vi "Sprinkler.vi"() -> ()   [LabVIEW 2013]
uses:
  Controls/Sprinkler State.ctl
  Controls/Read Write States.ctl
panel:
  in  "Zone Setup Array":cluster{"Zone Selector":string, "Timing":dbl}[](array[cluster])
  out "Controller Status":string
  out "Zone Indicators":T1
  in  "Water Pressure Sensor (%)":u32(slide) scale=0.0..100.0
  in  "Rain Sensor":bool
  in  "Run Selector":bool
  in  "Setup":bool
  in  "Start":bool
  in  "stop":bool
  # "Controls"
  # "Simulation Controls"
  # "Rain"
  # "No Rain"
  # "Continuous"
  # "Single"
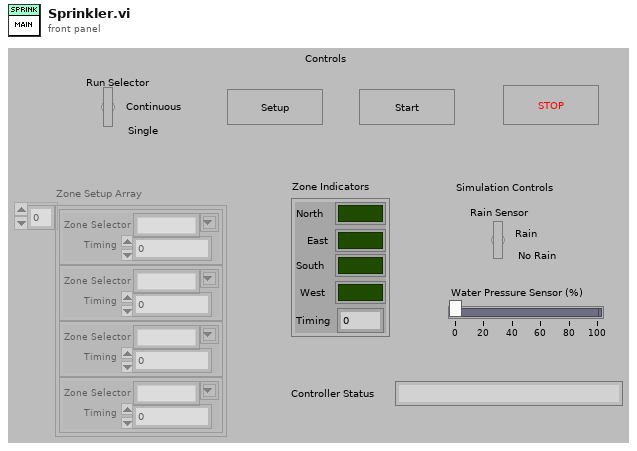
[diagram p1: front panel]
types:
  T1 = cluster{"North":bool, "East":bool, "South":bool, "West":bool, "Timing":u32}
  T2 = typedef "Sprinkler State.ctl" = enum16{"Initialize", "Main", "Stop"}
  T3 = enum8{"Enabled", "Disabled", "Disabled and Grayed Out"}
  T4 = typedef "Read Write States.ctl" = enum16{"Initialize", "Read", "Write", "Stop"}
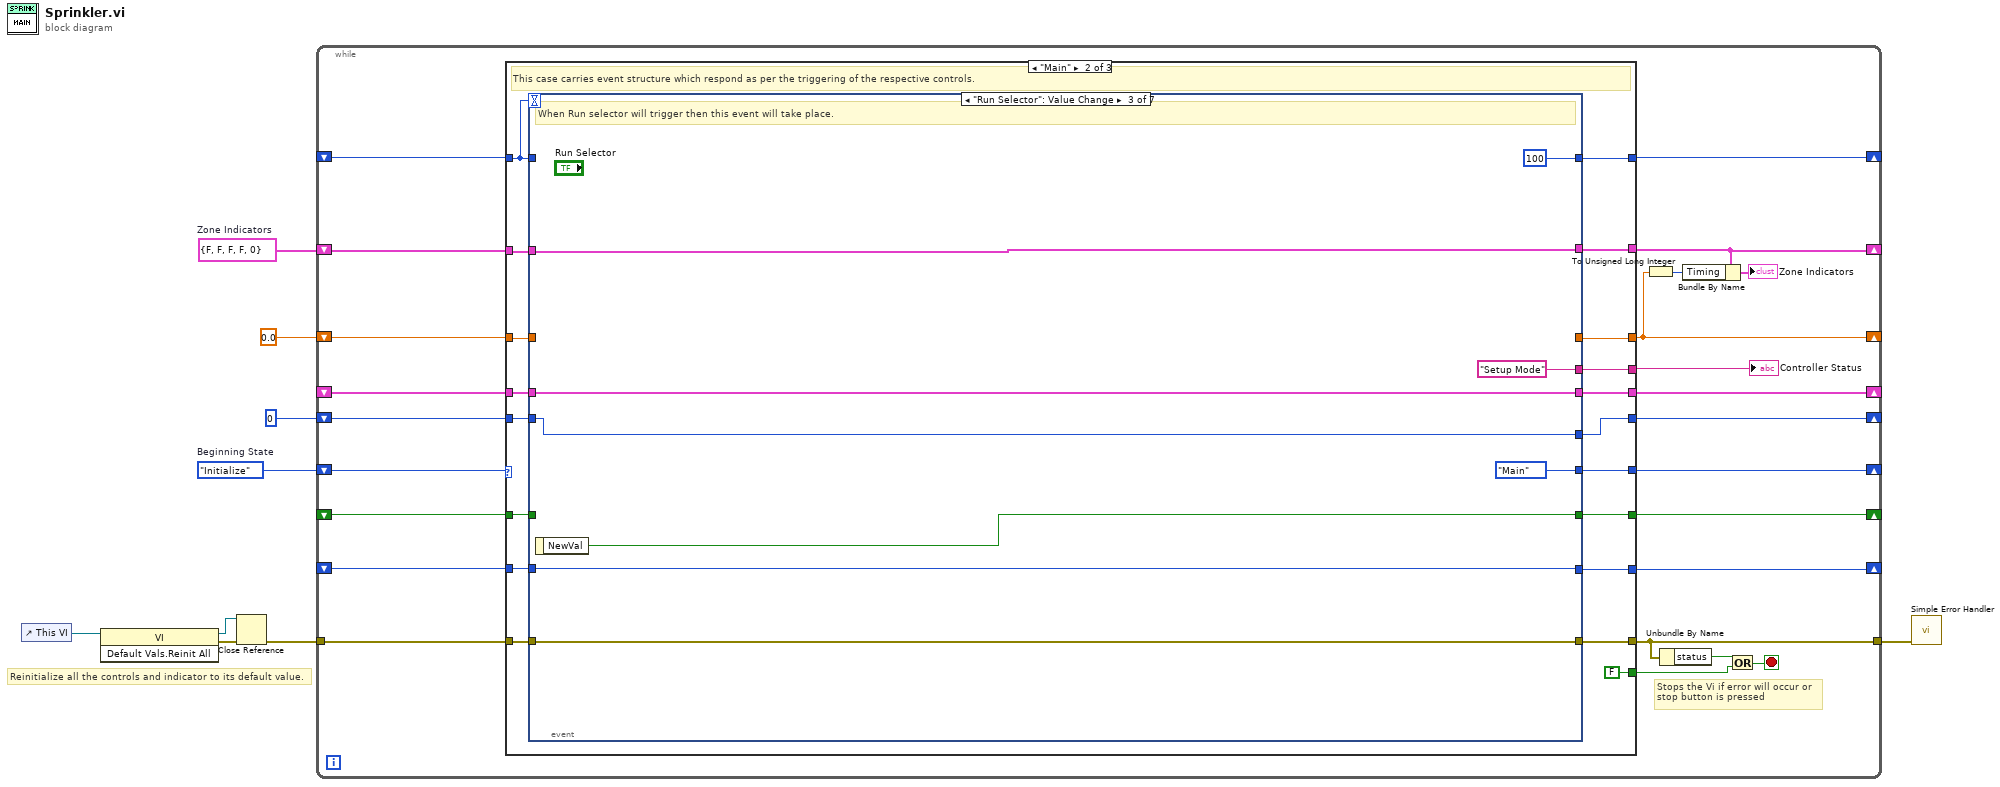
[diagram p0: block diagram]
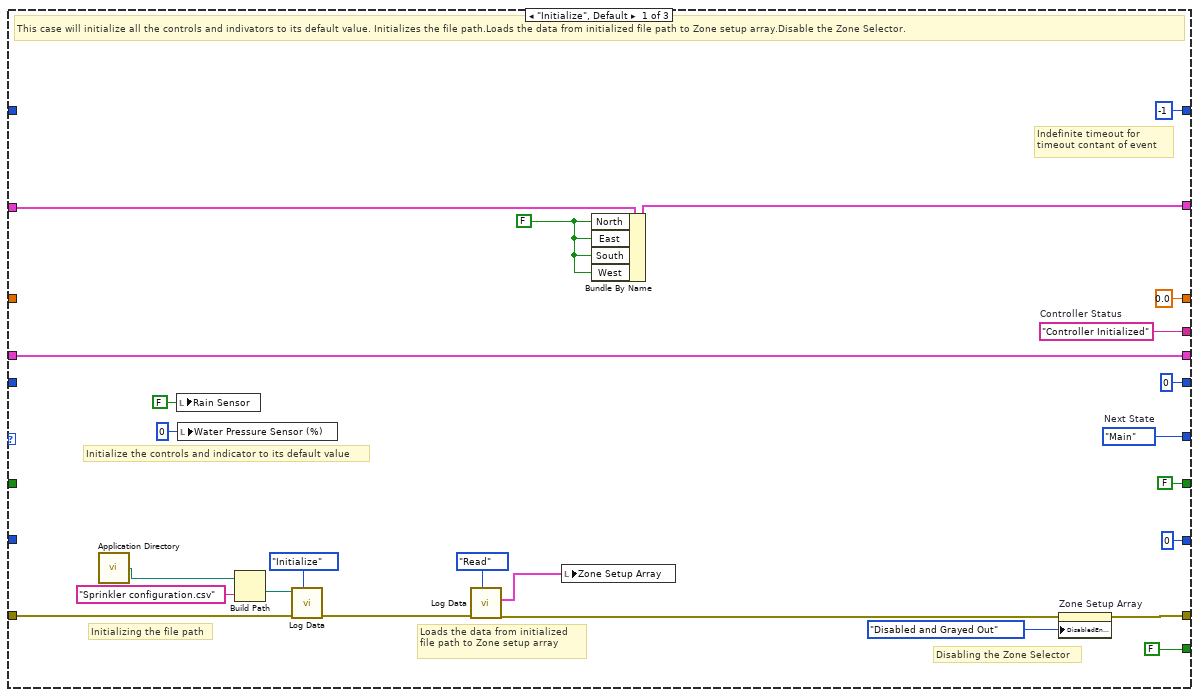
[diagram p2: hidden frame]
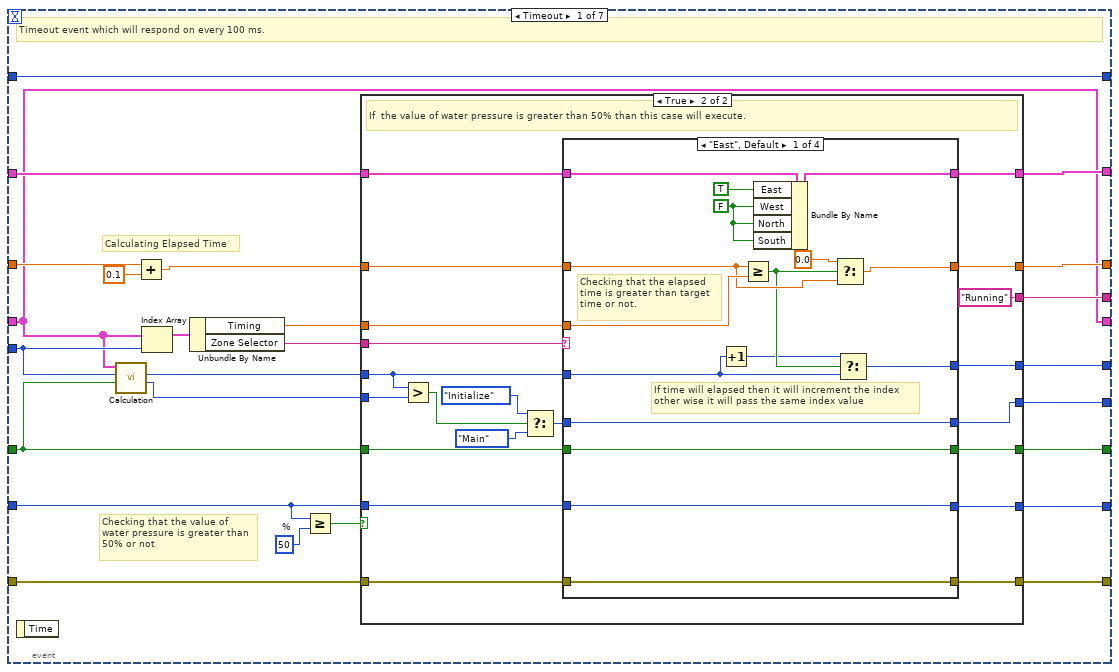
[diagram p3: hidden frame]
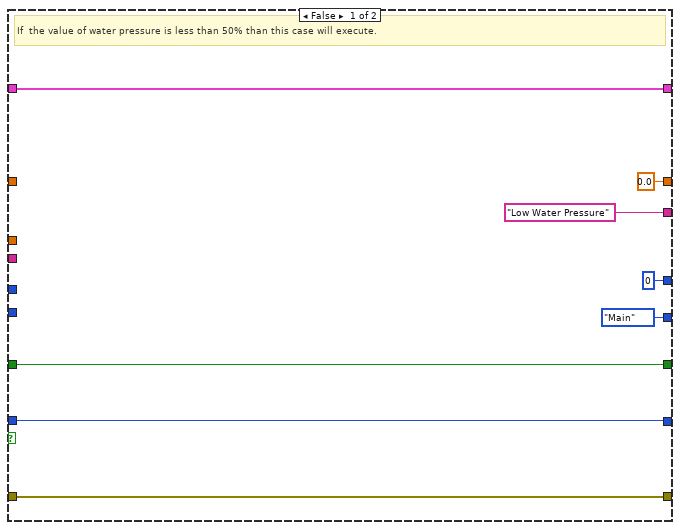
[diagram p4: hidden frame]
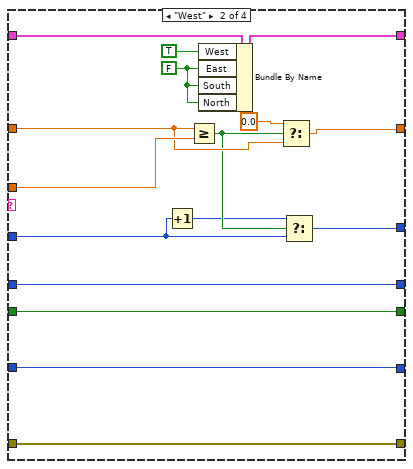
[diagram p5: hidden frame]
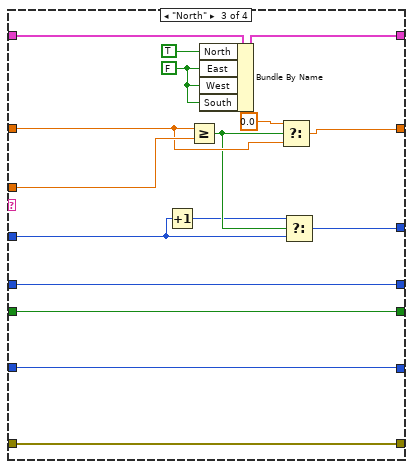
[diagram p6: hidden frame]
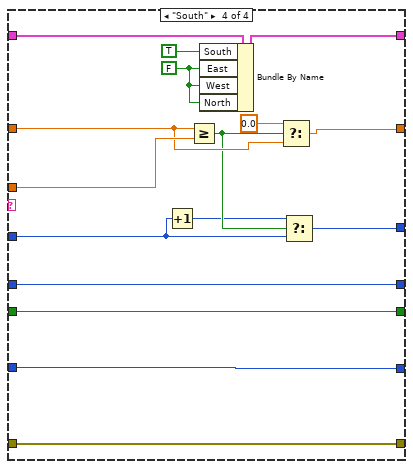
[diagram p7: hidden frame]
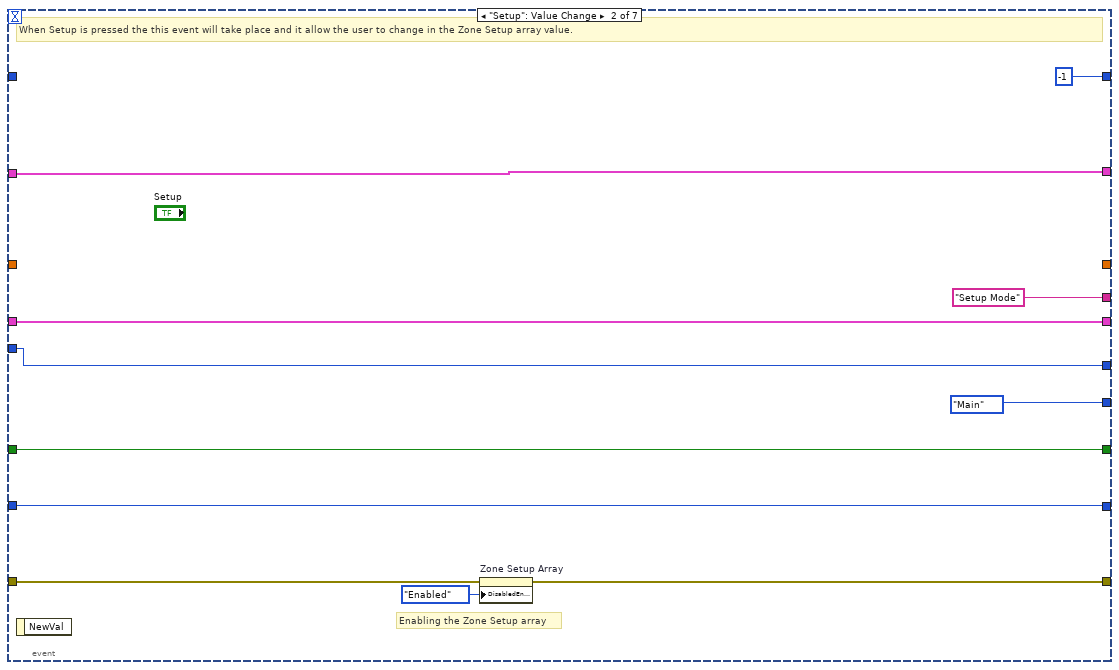
[diagram p8: hidden frame]
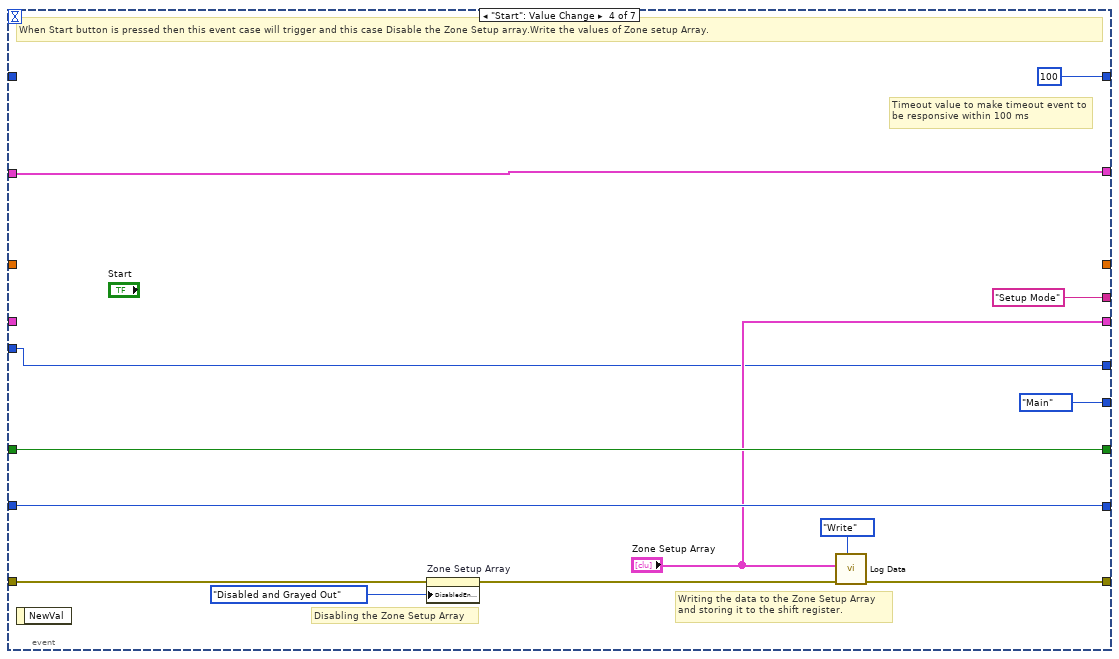
[diagram p9: hidden frame]
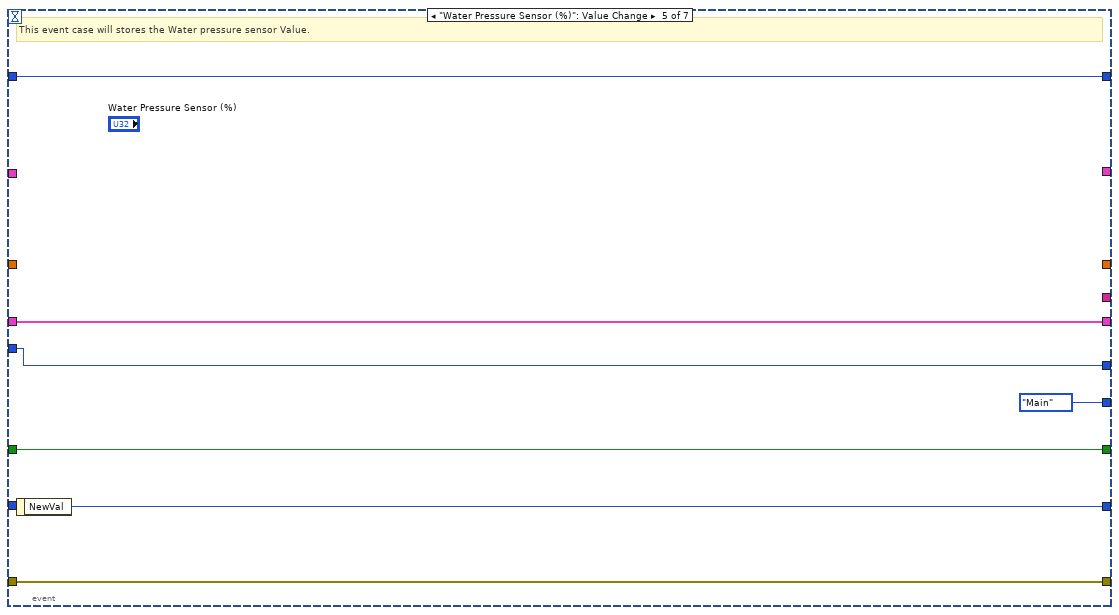
[diagram p10: hidden frame]
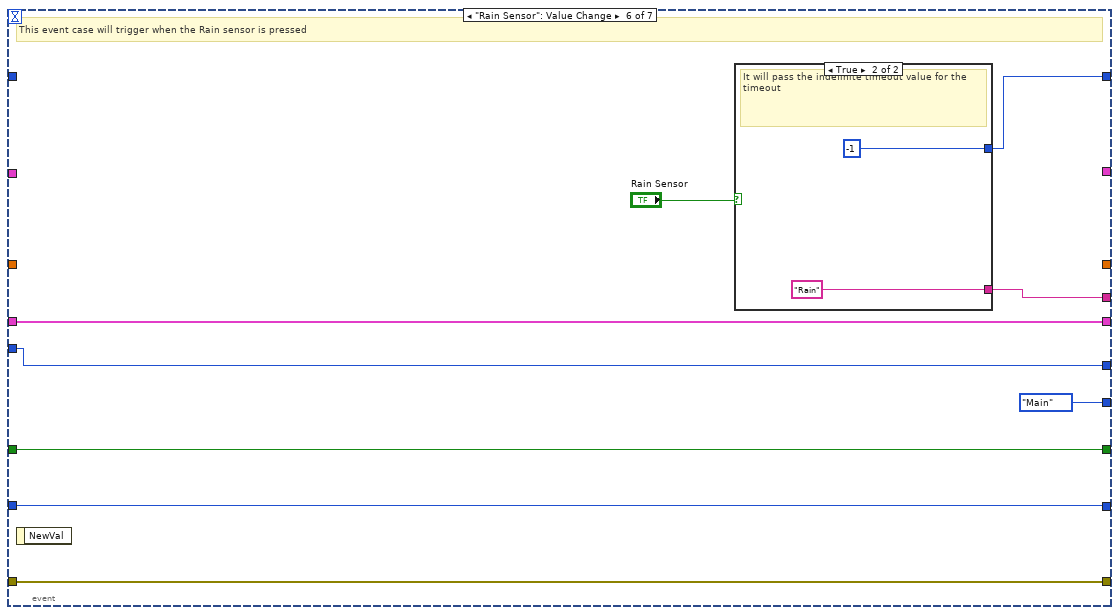
[diagram p11: hidden frame]
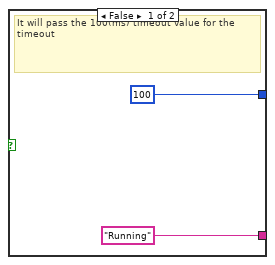
[diagram p12: hidden frame]
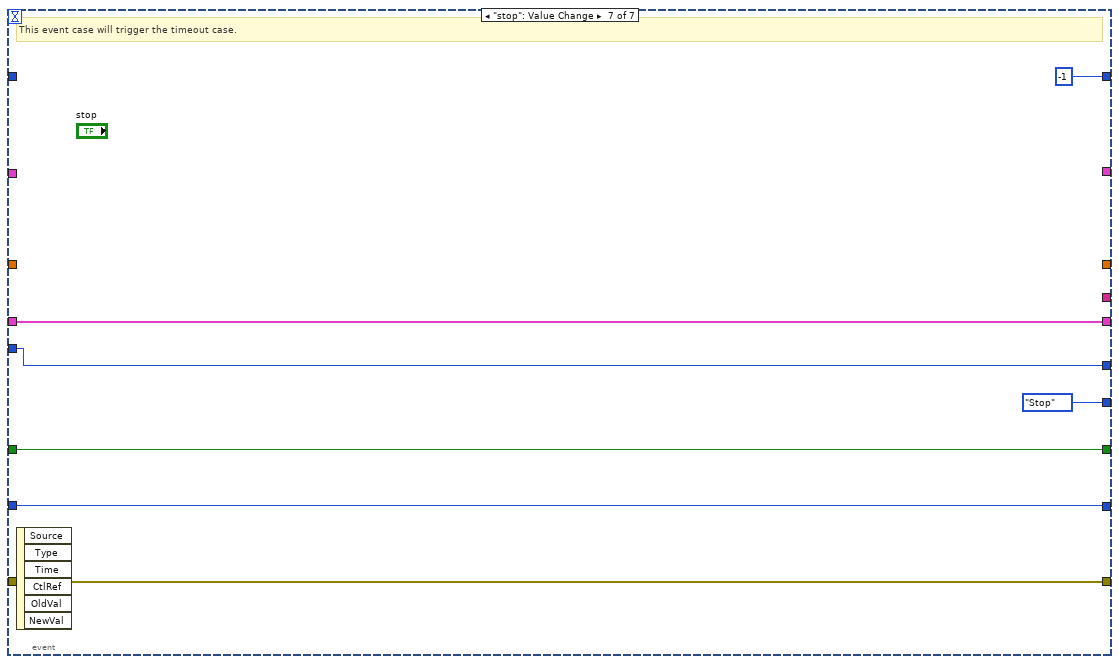
[diagram p13: hidden frame]
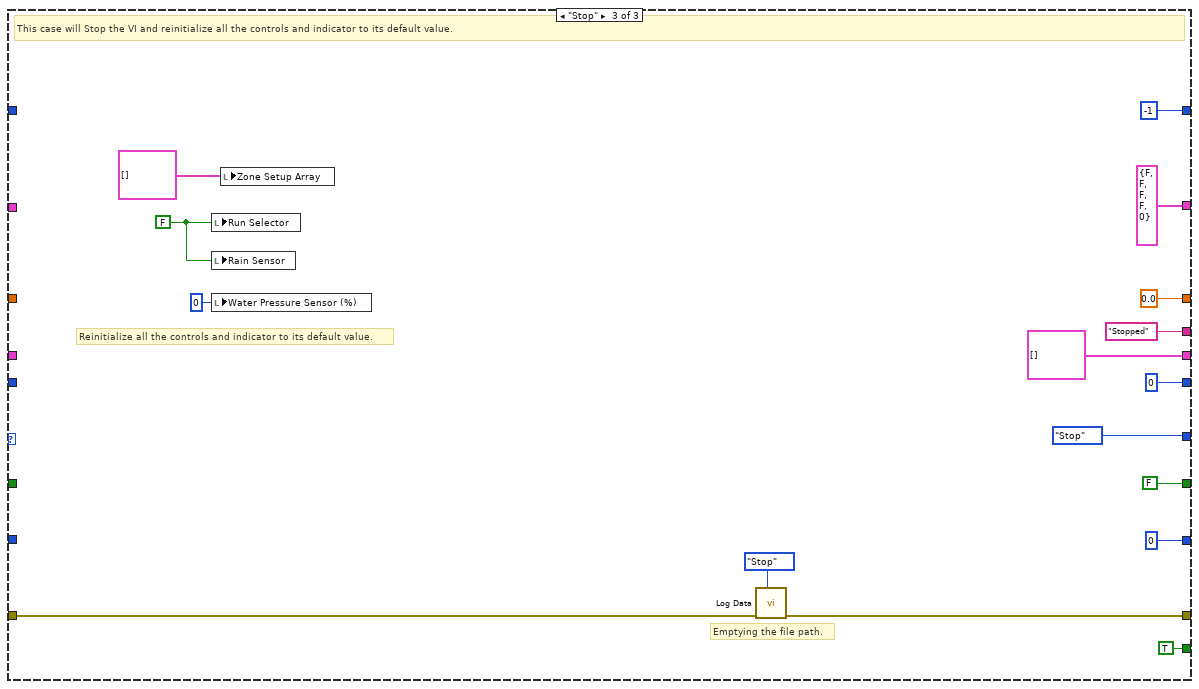
[diagram p14: hidden frame]
diagram:
  w4 = T1 {"North"=FALSE, "East"=FALSE, "South"=FALSE, "West"=FALSE, "Timing"=0}  # Zone Indicators
  w9 = Sprinkler_State."Initialize"  # Beginning State
  # "Reinitialize all the controls and indicator to its default value."
  n1 = control-ref of="This VI"() -> (w6:refnum<vi>)
  n2 = invoke class="VI" method="Default Vals.Reinit All"(reference=w6) -> (reference out=w7:refnum<vi>, error out=w8:errorcluster)  [unwired: 2 in, 1 out]
  n3 = Close Reference(reference=w7, error in (no error)=w8) -> (error out=w5:errorcluster)
  n4 = while {
    shift-right: [w32] -> _
    shift-left: w9 -> [w33]
    tunnel: w5 -> [w31]
    tunnel: [w27] -> w1
    shift-right: [w28] -> _
    shift-left: w4 -> [w29]
    shift-right: [w23] -> _
    shift-left: _ -> [w13]
    shift-right: [w22] -> _
    shift-left: _ -> [w21]
    shift-right: [w18] -> _
    shift-left: 0.0 -> [w20]
    shift-right: [w16] -> _
    shift-left: _ -> [w10]
    shift-right: [w14] -> _
    shift-left: 0 -> [w15]
    shift-right: [w12] -> _
    shift-left: _ -> [w11]
    stop <- w24 stop-if-true
    # "Stops the Vi if error will occur or stop button is pressed"
    n5 = case shown="\"Main\"" w33 {
      tunnel: [w58 w62 Sprinkler_State."Stop" ("Next State")] -> w32
      tunnel: w31 -> [w57 w76 w258]
      tunnel: [w39 w75 w257] -> w27
      tunnel: [w50 w74 "Stopped" ("Controller Status")] -> w30
      tunnel: [w36 w72 T1 {"North"=FALSE, "East"=FALSE, "South"=FALSE, "West"=FALSE, "Timing"=0} ("Zone Indicators")] -> w28
      tunnel: w29 -> [w49 w73 _]
      tunnel: [FALSE FALSE TRUE] -> w25
      tunnel: [FALSE ("NewVal") w71 FALSE ("NewVal")] -> w23
      tunnel: [-1 w70 -1] -> w22
      tunnel: w21 -> [_ w63 _]
      tunnel: w20 -> [_ w69 _]
      tunnel: [0.0 ("t") w68 0.0 ("t")] -> w18
      tunnel: [u32 0 ("NewVal") w67 u32 0 ("NewVal")] -> w16
      tunnel: w15 -> [_ w66 _]
      tunnel: [0 ("t") w65 0 ("t")] -> w14
      tunnel: w13 -> [_ w64 _]
      tunnel: [w37 w61 cluster{"Zone Selector":string, "Timing":dbl}[] [] ("Zone Setup Array")] -> w12
      tunnel: w11 -> [w37 w60 _]
      tunnel: w10 -> [_ w59 _]
      frame "Initialize", Default {
        w35 = FALSE ("North")
        w50 = "Controller Initialized"  # Controller Status
        w58 = Sprinkler_State."Main"  # Next State
        # "Indefinite timeout for \ntimeout contant of event"
        # "Disabling the Zone Selector"
        # "Loads the data from initialized file path to Zone setup array"
        # "Initializing the file path"
        # "Initialize the controls and indicator to its default value"
        # "This case will initialize all the controls and indivators to its default value. Initializes the file path.Loads the data from initialized file path to Zone setup array.Disable the Zone Selector."
        n6 = call <vilib>:"Application Directory.vi"() -> ("Application Directory"=w55:path)
        n7 = local write "Rain Sensor"(FALSE ("Rain Sensor")) -> ()
        n8 = local write "Water Pressure Sensor (%)"(u32 0 ("Water Pressure Sensor (%)")) -> ()
        n9 = Build Path(base path=w55, name or relative path="Sprinkler configuration.csv") -> (appended path=w53:path)
        n10 = call "Log Data.vi"("Command"=Read_Write_States."Initialize", "error in (no error)"=w57, "file path"=w53) -> ("error out"=w52:errorcluster)  [unwired: 7 in, 1 out]
        n11 = call "Log Data.vi"("Command"=Read_Write_States."Read", "error in (no error)"=w52) -> ("error out"=w40:errorcluster, "Array"=w38:cluster{"Zone Selector":string, "Timing":dbl}[])  [unwired: 8 in]
        n12 = local write "Zone Setup Array"(w38) -> ()
        n13 = Bundle By Name(cluster=w49, "North"=w35, "East"=w35, "South"=w35, "West"=w35) -> (w36:T1)
        n14 = property on="Zone Setup Array" class="Arr (strict)"(error in=w40, "DisabledEnum"=T3."Disabled and Grayed Out" ("Disabled")) -> (error out=w39:errorcluster)  [unwired: 1 in, 1 out]
      }
      frame "Main" {
        # "This case carries event structure which respond as per the triggering of the respective controls."
        n15 = event shown="[2] \"Run Selector\": Value Change" {
          selector: _ -> [_ _ _ _ _ _ _]
          dyn-events: _ -> [_ _ _ _ _ _ _]
          timeout: w63 -> [_ _ _ _ _ _ _]
          tunnel: w76 -> [w99 w199 w215 w223 w235 w244 w255]
          tunnel: [w98 w198 w215 w219 w235 w244 w255] -> w75
          tunnel: [w86 "Setup Mode" "Setup Mode" "Setup Mode" _ w237 _] -> w74
          tunnel: w73 -> [w94 w205 w214 w227 _ _ _]
          tunnel: [w93 w205 w214 w227 _ _ _] -> w72
          tunnel: [w84 w203 w213 w225 w233 w243 w254] -> w71
          tunnel: [w89 -1 100 100 w230 w238 -1] -> w70
          tunnel: w69 -> [w102 _ _ _ _ _ _]
          tunnel: [w96 _ _ _ _ _ _] -> w68
          tunnel: [w83 w197 w209 w221 w234 w240 w251] -> w67
          tunnel: w66 -> [w90 w196 w207 w216 w229 w236 w249]
          tunnel: [w92 w196 w207 w216 w229 w236 w249] -> w65
          tunnel: w64 -> [w85 w203 _ w225 w233 w243 w254]
          tunnel: w63 -> [w89 _ _ _ w230 _ _]
          tunnel: [w81 Sprinkler_State."Main" ("Next State") Sprinkler_State."Main" ("Next State") Sprinkler_State."Main" ("Next State") Sprinkler_State."Main" ("Next State") Sprinkler_State."Main" ("Next State") Sprinkler_State."Stop" ("Next State")] -> w62
          tunnel: [w80 w200 w211 "Zone Setup Array" w232 w242 w253] -> w61
          tunnel: w60 -> [w80 w200 w211 _ w232 w242 w253]
          tunnel: w59 -> [w82 w197 w209 w221 _ w240 w251]
          event Timeout {
            w88 = u32 50  # %
            # "Checking that the value of\nwater pressure is greater than\n50% or not"
            # "Calculating Elapsed Time"
            # "Timeout event which will respond on every 100 ms."
            n16 = event-data() -> ()  [unwired: 1 in, 1 out]
            n17 = call "Calculation.vi"("Zone Selector"=w85, "Index in"=w90, "Zone Setup Array"=w80) -> (1:"Index out"=w78:i32, 2:"Index out"=w79:i32)  [unwired: 6 in, 1 out]
            n18 = Add(x=w102, y=0.1) -> (x+y=w97:dbl)
            n19 = Index Array(array=w80, index=w90) -> (element=w100:cluster{"Zone Selector":string, "Timing":dbl})
            n20 = Unbundle By Name(w100) -> ("Timing"=w91:dbl, "Zone Selector"=w95:string)
            n21 = Greater Or Equal?(x=w82, y=w88) -> (x >= y?=w87:bool)
            n22 = case shown="True" w87 {
              tunnel: w99 -> [w105 w131]
              tunnel: [w105 w130] -> w98
              tunnel: w97 -> [_ w129]
              tunnel: [0.0 ("t") w128] -> w96
              tunnel: w95 -> [_ w127]
              tunnel: w94 -> [w109 w126]
              tunnel: [w109 w125] -> w93
              tunnel: [0 ("t") w118] -> w92
              tunnel: w91 -> [_ w124]
              tunnel: w79 -> [_ w117]
              tunnel: ["Low Water Pressure" "Running"] -> w86
              tunnel: w85 -> [w106 w121]
              tunnel: [w106 w122] -> w84
              tunnel: [w104 w120] -> w83
              tunnel: w82 -> [w104 w119]
              tunnel: [Sprinkler_State."Main" ("Next State") w112] -> w81
              tunnel: w78 -> [_ w111]
              frame False {
                # "If  the value of water pressure is less than 50% than this case will execute."
              }
              frame True {
                # "If  the value of water pressure is greater than 50% than this case will execute."
                n23 = Greater?(x=w117, y=w111) -> (0:w116:bool)
                n24 = Select(t=Sprinkler_State."Initialize" ("Next State"), s=w116, f=Sprinkler_State."Main" ("Next State")) -> (s? t:f=w113:T2)
                n25 = case shown="\"East\", Default" w127 {
                  tunnel: w131 -> [w147 w163 w179 w195]
                  tunnel: [w147 w163 w179 w195] -> w130
                  tunnel: w129 -> [w142 w158 w174 w190]
                  tunnel: [w140 w156 w172 w188] -> w128
                  tunnel: w126 -> [w146 w162 w178 w194]
                  tunnel: [w145 w161 w177 w193] -> w125
                  tunnel: [w138 w154 w170 w186] -> w118
                  tunnel: w124 -> [w143 w159 w175 w191]
                  tunnel: w117 -> [w136 w152 w168 w184]
                  tunnel: [w134 w150 w166 w182] -> w122
                  tunnel: w121 -> [w134 w150 w166 w182]
                  tunnel: [w133 w149 w165 w181] -> w120
                  tunnel: w119 -> [w133 w149 w165 w181]
                  tunnel: w113 -> [w132 w148 w164 w180]
                  tunnel: [w132 w148 w164 w180] -> w112
                  frame "East", Default {
                    w135 = FALSE ("South")
                    # "If time will elapsed then it will increment the index\nother wise it will pass the same index value"
                    # "Checking that the elapsed \ntime is greater than target \ntime or not."
                    n26 = Increment(x=w136) -> (x+1=w137:i32)
                    n27 = Greater Or Equal?(x=w142, y=w143) -> (x >= y?=w139:bool)
                    n28 = Bundle By Name(cluster=w146, "East"=TRUE, "West"=w135, "North"=w135, "South"=w135) -> (w145:T1)
                    n29 = Select(t=0.0, s=w139, f=w142) -> (s? t:f=w140:dbl)
                    n30 = Select(t=w137, s=w139, f=w136) -> (s? t:f=w138:i32)
                  }
                  frame "West" {
                    w151 = FALSE ("West")
                    n31 = Increment(x=w152) -> (x+1=w153:i32)
                    n32 = Greater Or Equal?(x=w158, y=w159) -> (x >= y?=w155:bool)
                    n33 = Bundle By Name(cluster=w162, "West"=TRUE ("East"), "East"=w151, "South"=w151, "North"=w151) -> (w161:T1)
                    n34 = Select(t=0.0, s=w155, f=w158) -> (s? t:f=w156:dbl)
                    n35 = Select(t=w153, s=w155, f=w152) -> (s? t:f=w154:i32)
                  }
                  frame "North" {
                    w167 = FALSE ("West")
                    n36 = Increment(x=w168) -> (x+1=w169:i32)
                    n37 = Greater Or Equal?(x=w174, y=w175) -> (x >= y?=w171:bool)
                    n38 = Bundle By Name(cluster=w178, "North"=TRUE ("East"), "East"=w167, "West"=w167, "South"=w167) -> (w177:T1)
                    n39 = Select(t=0.0, s=w171, f=w174) -> (s? t:f=w172:dbl)
                    n40 = Select(t=w169, s=w171, f=w168) -> (s? t:f=w170:i32)
                  }
                  frame "South" {
                    w183 = FALSE ("West")
                    n41 = Increment(x=w184) -> (x+1=w185:i32)
                    n42 = Greater Or Equal?(x=w190, y=w191) -> (x >= y?=w187:bool)
                    n43 = Bundle By Name(cluster=w194, "South"=TRUE ("East"), "East"=w183, "West"=w183, "North"=w183) -> (w193:T1)
                    n44 = Select(t=0.0, s=w187, f=w190) -> (s? t:f=w188:dbl)
                    n45 = Select(t=w185, s=w187, f=w184) -> (s? t:f=w186:i32)
                  }
                }
              }
            }
          }
          event "Setup": Value Change {
            # "Enabling the Zone Setup array"
            # "When Setup is pressed the this event will take place and it allow the user to change in the Zone Setup array value."
            n46 = event-data() -> ()  [unwired: 1 in, 1 out]
            n47 = property on="Zone Setup Array" class="Arr (strict)"(error in=w199, "DisabledEnum"=T3."Enabled" ("Disabled")) -> (error out=w198:errorcluster)  [unwired: 1 in, 1 out]
          }
          event "Run Selector": Value Change {
            # "When Run selector will trigger then this event will take place."
            n48 = event-data() -> ("NewVal"=w213:bool)  [unwired: 1 in]
          }
          event "Start": Value Change {
            # "Timeout value to make timeout event to be responsive within 100 ms"
            # "Writing the data to the Zone Setup Array\nand storing it to the shift register."
            # "Disabling the Zone Setup Array"
            # "When Start button is pressed then this event case will trigger and this case Disable the Zone Setup array.Write the values of Zone setup Array."
            n49 = event-data() -> ()  [unwired: 1 in, 1 out]
            n50 = property on="Zone Setup Array" class="Arr (strict)"(error in=w223, "DisabledEnum"=T3."Disabled and Grayed Out" ("Disabled")) -> (error out=w220:errorcluster)  [unwired: 1 in, 1 out]
            n51 = call "Log Data.vi"("Command"=Read_Write_States."Write", "error in (no error)"=w220, "Zone Setup Array"="Zone Setup Array") -> ("error out"=w219:errorcluster)  [unwired: 7 in, 1 out]
          }
          event "Water Pressure Sensor (%)": Value Change {
            # "This event case will stores the Water pressure sensor Value."
            n52 = event-data() -> ("NewVal"=w234:u32)  [unwired: 1 in]
          }
          event "Rain Sensor": Value Change {
            # "This event case will trigger when the Rain sensor is pressed"
            n53 = event-data() -> ()  [unwired: 1 in, 1 out]
            n54 = case shown="True" "Rain Sensor" {
              tunnel: ["Running" "Rain"] -> w237
              tunnel: [100 -1] -> w238
              frame False {
                # "It will pass the 100(ms) timeout value for the timeout"
              }
              frame True {
                # "It will pass the indefinite timeout value for the timeout"
              }
            }
          }
          event "stop": Value Change {
            # "This event case will trigger the timeout case."
            n55 = event-data() -> ()  [unwired: 1 in, 6 out]
          }
        }
      }
      frame "Stop" {
        w259 = FALSE ("Run Selector")
        # "Emptying the file path."
        # "Reinitialize all the controls and indicator to its default value."
        # "This case will Stop the VI and reinitialize all the controls and indicator to its default value."
        n56 = local write "Run Selector"(w259) -> ()
        n57 = local write "Rain Sensor"(w259) -> ()
        n58 = local write "Water Pressure Sensor (%)"(u32 0 ("Water Pressure Sensor (%)")) -> ()
        n59 = local write "Zone Setup Array"(cluster{"Zone Selector":string, "Timing":dbl}[] [] ("Zone Setup Array")) -> ()
        n60 = call "Log Data.vi"("Command"=Read_Write_States."Stop", "error in (no error)"=w258) -> ("error out"=w257:errorcluster)  [unwired: 8 in, 1 out]
      }
    }
    "Controller Status" <- w30
    n61 = To Unsigned Long Integer(number=w18) -> (unsigned 32bit integer=w17:u32)
    n62 = Unbundle By Name(w27) -> ("status"=w26:bool)
    n63 = Bundle By Name(cluster=w28, "Timing"=w17) -> (→"Zone Indicators":T1)
    n64 = Or(x=w26, y=w25) -> (x .or. y?=w24:bool)
  }
  n65 = call <vilib>:"Simple Error Handler.vi"("error in (no error)"=w1) -> ()  [unwired: 4 in, 5 out]
